vi "ImClass_Read_Dataset_All.vi"(6 "Dims(C,H,W)":T1={"C"=-1, "H"=-1, "W"=-1}, 8 "error in (no error)":errorcluster, 10 "Test Path":path, 11 "Train Path":path) -> (0 "error out":errorcluster, 3 "Dataset":T2={"Train"={"Inputs Ref."=variant(refnum<data-value> refnum), "Outputs Ref."=refnum, "Dataset_Size"=0, "Dims_In"={"C"=0, "H"=0, "W"=0}, "Dims_Out"=0, "Labels"=[], "File Paths"=[], "Custom_Data"=variant}, "Validation"={"Inputs Ref."=variant(refnum<data-value> refnum), "Outputs Ref."=refnum, "Dataset_Size"=0, "Dims_In"={"C"=0, "H"=0, "W"=0}, "Dims_Out"=0, "Labels"=[], "File Paths"=[], "Custom_Data"=variant}, "Test"={"Inputs Ref."=variant(refnum<data-value> refnum), "Outputs Ref."=refnum, "Dataset_Size"=0, "Dims_In"={"C"=0, "H"=0, "W"=0}, "Dims_Out"=0, "Labels"=[], "File Paths"=[], "Custom_Data"=variant}})   [LabVIEW 2020]
uses:
  <vilib>/Ngene/Deep Learning Toolkit/Toolkit/NN_Data/API/DataSet/DataSet_Types/NN_DataSets_All(In3D_Out1D).ctl
  <vilib>/Ngene/Deep Learning Toolkit/Toolkit/NN_Data/API/DataSet/DataSet_Types/NN_DataSet(In3D_Out1D).ctl
  <vilib>/Ngene/Deep Learning Toolkit/Toolkit/NN_Data/Controls/DataRef_Types/2D/NN_Data_ref(2D_SGL).ctl
  <vilib>/Ngene/Deep Learning Toolkit/Toolkit/NN_Data/API/NN_Dims(C,H,W).ctl
  <vilib>/Ngene/Deep Learning Toolkit/Toolkit/Deep_Learning_Toolkit_by_Ngene.lvlib
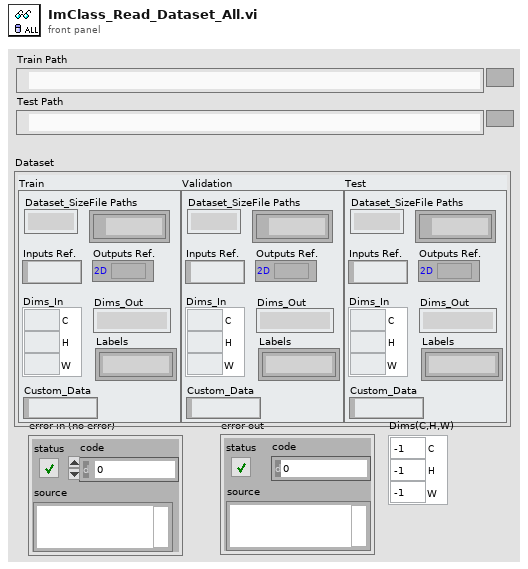
[diagram p1: front panel]
types:
  T1 = typedef "Deep_Learning_Toolkit_by_Ngene.lvlib/NN_Dims(C,H,W).ctl" = cluster{"C":i32, "H":i32, "W":i32}
  T2 = typedef "Deep_Learning_Toolkit_by_Ngene.lvlib/NN_DataSets_All(In3D_Out1D).ctl" = cluster{"Train":T3, "Validation":T3, "Test":T3}
  T3 = typedef "Deep_Learning_Toolkit_by_Ngene.lvlib/NN_DataSet(In3D_Out1D).ctl" = cluster{"Inputs Ref.":variant, "Outputs Ref.":T4, "Dataset_Size":i32, "Dims_In":T1, "Dims_Out":i32, "Labels":string[], "File Paths":path[], "Custom_Data":variant}
  T4 = typedef "Deep_Learning_Toolkit_by_Ngene.lvlib/NN_Data_ref(2D_SGL).ctl" = refnum<data-value>
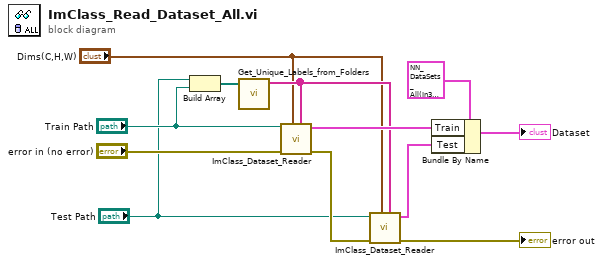
[diagram p0: block diagram]
diagram:
  n1 = Build Array("Test Path", "Train Path") -> (w5:path[])
  n2 = call "Get_Unique_Labels_from_Folders.vi"("Folder Path"=w5) -> ("Unique_Folders"=w2:string[])  [unwired: 9 in, 1 out]
  n3 = call "ImClass_Dataset_Reader.vi"("Unique labels"=w2, "Dims(C,H,W)"="Dims(C,H,W)", "error in (no error)"="error in (no error)", "Image Foldr Path"="Train Path") -> ("error out"=w10:errorcluster, "NN_DataSet(In3D_OutBBox)"=w11:T3)  [unwired: 6 in]
  n4 = call "ImClass_Dataset_Reader.vi"("Unique labels"=w2, "Dims(C,H,W)"="Dims(C,H,W)", "error in (no error)"=w10, "Image Foldr Path"="Test Path") -> ("error out"=→"error out":errorcluster, "NN_DataSet(In3D_OutBBox)"=w3:T3)  [unwired: 6 in]
  n5 = Bundle By Name(cluster=T2 {"Train"={"Inputs Ref."=variant(refnum<data-value> refnum), "Outputs Ref."=refnum, "Dataset_Size"=0, "Dims_In"={"C"=0, "H"=0, "W"=0}, "Dims_Out"=0, "Labels"=[], "File Paths"=[], "Custom_Data"=variant}, "Validation"={"Inputs Ref."=variant(refnum<data-value> refnum), "Outputs Ref."=refnum, "Dataset_Size"=0, "Dims_In"={"C"=0, "H"=0, "W"=0}, "Dims_Out"=0, "Labels"=[], "File Paths"=[], "Custom_Data"=variant}, "Test"={"Inputs Ref."=variant(refnum<data-value> refnum), "Outputs Ref."=refnum, "Dataset_Size"=0, "Dims_In"={"C"=0, "H"=0, "W"=0}, "Dims_Out"=0, "Labels"=[], "File Paths"=[], "Custom_Data"=variant}} ("Datasets_All(In3D_Out1D)"), "Train"=w11, "Test"=w3) -> (→"Dataset":T2)
